vi "BuildCommand_InvokePPP.vi"(8 "error in (no error)":errorcluster, 11 "Cluster":T49 {"PersistentData"."RecircPumpFlow"."Recirc Pump Flow Set - R6" min=0.0 max=20.0; "PersistentData"."RecircPumpFlow"."Recirc Pump Flow Set - R5" min=0.0 max=20.0; "PersistentData"."RecircPumpFlow"."Recirc Pump Flow Set - R4" min=0.0 max=20.0; "PersistentData"."RecircPumpFlow"."Recirc Pump Flow Set - R3" min=0.0 max=20.0; "PersistentData"."RecircPumpFlow"."Recirc Pump Flow Set - R2" min=0.0 max=20.0; "PersistentData"."RecircPumpFlow"."Recirc Pump Flow Set - R1" min=0.0 max=20.0; "PersistentData"."MiniscusPressure"."Meniscus Pressure Set - R6" min=0.0 max=20.0; "PersistentData"."MiniscusPressure"."Meniscus Pressure Set - R5" min=0.0 max=20.0; "PersistentData"."MiniscusPressure"."Meniscus Pressure Set - R4" min=0.0 max=20.0; "PersistentData"."MiniscusPressure"."Meniscus Pressure Set - R3" min=0.0 max=20.0; "PersistentData"."MiniscusPressure"."Meniscus Pressure Set - R2" min=0.0 max=20.0; "PersistentData"."MiniscusPressure"."Meniscus Pressure Set - R1" min=0.0 max=20.0; "PersistentData"."Meniscus Vac Pump Speed" min=0.0 max=100.0}) -> (0 "error out":errorcluster, 2 "NextState":string, 3 "PPP Dithered Images":path[](array[path]))   [LabVIEW 2022 SP3, in "TopLevel.lvclass"]
uses:
  TopLevel.lvclass
  IO/IO.lvclass
  GIS Printer/GIS Printer.lvclass
  Motor Controller/Motor Controller.lvclass
  Typedefs/Digilens Config Cluster.ctl
  Typedefs/Motor Controller Config Data.ctl
  IO/Typedefs/IO Config Data.ctl
  IO/Typedefs/DCON_DeviceConfig--Cluster.ctl
  IO/Typedefs/Channel Data.ctl
  GIS Printer/Typedefs/PrinterConfiguration--Cluster.ctl
  DAQWFE/LV_Source/Subsystems/DAQ/DataTypes/TD DAQ Settings--cluster.ctl
  DAQWFE/LV_Source/Subsystems/DAQ/DataTypes/TD DI Instrument Settings--cluster.ctl
  DAQWFE/LV_Source/Subsystems/DAQ/DataTypes/TD AI Instrument Settings--cluster.ctl
  DAQWFE/LV_Source/Subsystems/DAQ/DataTypes/TD AI InstSettings--cluster.ctl
  DAQWFE/LV_Source/Subsystems/DAQ/Process/ProcessSupport/TD SimAI Ranges--cluster.ctl
  Common/Controls/DLPConfig_Initialization.ctl
  DLP2/DataTypes/DLP2_PrinterCompensationProperties.ctl
  DLP2/DataTypes/DLP2_PrinterHeadProperties.ctl
  Common/Controls/DLPConfig)Init_HeadPropertyAttr--Cluster.ctl
  DLP2/DataTypes/DLP2_PrinterMaterialProperties.ctl
  Typedefs/InkIdleNodeConfigXML--Cluster.ctl
  Typedefs/InkProcessNodeConfigXML--Cluster.ctl
  Motor Controller/Typedefs/Status.ctl
  Motor Controller/Typedefs/Stage Move Data.ctl
  Motor Controller/Typedefs/Batch Index Speed Data.ctl
  Motor Controller/Typedefs/Move Status.ctl
  IO/Typedefs/ICP1-D0 Channel Names.ctl
  IO/Typedefs/Pre Purge Parameters.ctl
  Typedefs/API Command Enum.ctl
  Database/Database.lvclass
  DLP2/DLP2.lvclass
  Common/Controls/TD MasterConfiguration DLPC2--cluster.ctl
  Common/Controls/DLPC2_Path--Cluster.ctl
  Common/Controls/TD HeadColorPaneMappingAll--cluster.ctl
  Common/Controls/TD HeadColorPaneMapping--cluster.ctl
  Typedefs/SpitVoltages--Cluster.ctl
  Typedefs/PrimingMode APIData.ctl
  Typedefs/PurgeMode--Enum.ctl
  Typedefs/PrinterHeads--Enum.ctl
  Common/Controls/RecipeInfo--Cluster.ctl
  DAQWFE/LV_Source/Subsystems/DAQ/DAQ.lvclass
  <vilib>/vision/Image Controls.llb/IMAQ Image.ctl
  Typedefs/TiffImageData--Cluster.ctl
  Common/Controls/Imageresolution--cluster.ctl
  GIS Printer/Typedefs/GIS Status--Cluster.ctl
  GIS Printer/Typedefs/HeadEnableStatus--cluster.ctl
  <vilib>/TELLC/Dynamic CVT API/TD Dynamic CVT DVR--ref.ctl
  DLP2/DataTypes/SeperateLayersPython--cluster.ctl
  Common/Controls/PythonVersion--Enum.ctl
  Common/Controls/PersistentData--Cluster.ctl
  Common/Controls/DLPConfig_RecipePrints.ctl
  Common/Controls/DLPConfig_CalibrationPrints.ctl
  Typedefs/LoginEventData--CLuster.ctl
  Typedefs/UserLevel--Enum.ctl
  Typedefs/printWeights--cluster.ctl
  DLP2/DataTypes/PPP_Python--cluster.ctl
  Common/Controls/DLP_MaterialToHeadMapping--Cluster.ctl
types:
  T1 = typedef "TopLevel.lvclass/Digilens Config Cluster.ctl" = cluster{"Motion Controller":T2, "IO Config":T3, "PrinterConfiguration":T6, "DAQ Settings":T7}
  T2 = typedef "Motor Controller.lvclass/Motor Controller Config Data.ctl" = cluster{"Motor IP Addresss":string, "Current Position":i32, "Pulse_Per_mm":i32, "PrePrint":dbl[], "Load Position_mm":i32, "Laminate Position_mm":i32}
  T3 = typedef "IO.lvclass/IO Config Data.ctl" = cluster{"DAQDevices":T4[], "DI Channels":T5[], "DO Channels":T5[], "Material Names":string[], "AI Channels":T5[], "AO Channels":T5[]}
  T4 = typedef "IO.lvclass/DCON_DeviceConfig--Cluster.ctl" = cluster{"COM":string, "DeviceName":string, "BaudRate":u32, "Number of Channels":i32, "DeviceAddress":i32, "Enable":bool}
  T5 = typedef "IO.lvclass/Channel Data.ctl" = cluster{"Channel Name":string, "Device Name":string, "Channel No":string}
  T6 = typedef "GIS Printer.lvclass/PrinterConfiguration--Cluster.ctl" = cluster{"IPAddress":string, "Move Stage on RTP Command?":bool, "Stage Move Position":string, "PH1-Prime Path":path, "PH2-Prime Path":path, "PH3-Prime Path":path, "PH4-Prime Path":path, "PH5-Prime Path":path, "PH6-Prime Path":path, "PrintScriptsFolder":path, "PurgeScriptsFolder":path, "StageScriptsFolder":path, "PH1-HeatOn Path":path, "PH2-HeatOn Path":path, "PH3-HeatOn Path":path, "PH4-HeatOn Path":path, "PH5-HeatOn Path":path, "PH6-HeatOn Path":path, "PH1-HeatOff Path":path, "PH2-HeatOff Path":path, "PH3-HeatOff Path":path, "PH4-HeatOff Path":path, "PH5-HeatOff Path":path, "PH6-HeatOff Path":path}
  T7 = typedef "DAQ.lvclass/TD DAQ Settings--cluster.ctl" = cluster{"Simulate DAQ":bool, "DI Settings":T8[], "AI Settings":T9[], "Relay IONames":string[], "AO IONames":string[], "AO NChan SingleTask":bool}
  T8 = typedef "DAQ.lvclass/TD DI Instrument Settings--cluster.ctl" = cluster{"Disable":bool, "DI TaskName":string, "DI RefreshIntv":i32}
  T9 = typedef "DAQ.lvclass/TD AI Instrument Settings--cluster.ctl" = cluster{"Disable":bool, "AI TaskName":string, "AI InstSettings":T10, "SimAI Ranges":T11}
  T10 = typedef "DAQ.lvclass/TD AI InstSettings--cluster.ctl" = cluster{"DaqRate":dbl, "NumSamples":i32}
  T11 = typedef "DAQ.lvclass/TD SimAI Ranges--cluster.ctl" = cluster{"lo":dbl, "hi":dbl}
  T12 = typedef "DLPConfig_Initialization.ctl" = cluster{"PrinterInitialization":cluster{"Printer":cluster{"#attributes":cluster{"Name":string}}, "VacPumpSet":cluster{"#attributes":cluster{"VacPumpEnable":bool, "VacPumpSpeed":dbl}}, "HIBEnable":cluster{"#attributes":cluster{"HIB1Enable":bool, "HIB2Enable":bool, "HIB3Enable":bool, "HIB4Enable":bool, "HIB5Enable":bool, "HIB6Enable":bool}}, "PrinterCompensation":T13}, "HeadSet":cluster{"HeadProperties":T14[]}, "InkSet":cluster{"Ink":T16[]}, "Troubleshooting":cluster{"PMBLogging":cluster{"#attributes":cluster{"PMBMonitorDuringPrint":bool, "PMBMonitorDuringIdle":bool, "LogSwatheInputData":bool, "LogSwatheOutputData":bool, "LogPrintheadColourPlanes":bool, "LogPMBCommunication":bool, "LogSimulatedOutput":bool, "LogAllPMBCommunicationData":bool, "LogPMBSpace":bool, "ExtendedPMBSpaceLogging":bool, "LogPMBWriteSpeed":bool, "LogUsbRetries":bool}}, "HIBLogging":cluster{"#attributes":cluster{"HIBMonitoringDuringPrint":bool, "HIBMonitoringLog":bool}}}}
  T13 = typedef "DLP2_PrinterCompensationProperties.ctl" = cluster{"#attributes":cluster{"AppName":string, "PrintWeightMultiplier":dbl, "Rotation":bool, "Driver":string, "Server":string, "Database":string, "User":string, "Password":string}}
  T14 = typedef "DLP2_PrinterHeadProperties.ctl" = cluster{"#attributes":T15}
  T15 = typedef "DLPConfig)Init_HeadPropertyAttr--Cluster.ctl" = cluster{"HeadNumber":u8, "Material":string, "HeadLocalX":dbl, "HeadLocalY":dbl, "HeadRotationAngle":dbl, "VH2L_Hi":dbl, "VH2R_Hi":dbl, "VH1LA_Hi":dbl, "VH1LB_Hi":dbl, "VH1RA_Hi":dbl, "VH1RB_Hi":dbl, "VH2L_Lo":dbl, "VH2R_Lo":dbl, "VH1LA_Lo":dbl, "VH1LB_Lo":dbl, "VH1RA_Lo":dbl, "VH1RB_Lo":dbl}
  T16 = typedef "DLP2_PrinterMaterialProperties.ctl" = cluster{"#attributes":cluster{"InkType":string, "PrePrintPurge":bool, "PurgeTime":dbl, "PurgeCount":i32, "Density":dbl, "NumberofDrops":i32, "PrintWeight":dbl, "PrintheadPrime":bool}, "Idle":T17, "Process":T18}
  T17 = typedef "InkIdleNodeConfigXML--Cluster.ctl" = cluster{"ShortIdle":cluster{"#attributes":cluster{"Heat":dbl, "Meniscus":dbl, "Recirculation":bool}}, "LongIdle":cluster{"#attributes":cluster{"Heat":dbl, "Meniscus":dbl, "Recirculation":bool}}}
  T18 = typedef "InkProcessNodeConfigXML--Cluster.ctl" = cluster{"C30_Process":cluster{"#attributes":cluster{"Heat":dbl, "Meniscus":dbl, "Recirculation":bool, "ColorPlane":string}}, "S30_Process":cluster{"#attributes":cluster{"Heat":dbl, "Meniscus":dbl, "Recirculation":bool, "ColorPlane":string}}}
  T19 = typedef "Motor Controller.lvclass/Status.ctl" = cluster{"Motor Controller Config Data":T2, "Motor Controller Data":cluster{"Enabled?":bool}, "Stage Move":T20, "Stage Busy?":bool}
  T20 = typedef "Motor Controller.lvclass/Stage Move Data.ctl" = cluster{"Current Step":string, "Move Data":T21[]}
  T21 = typedef "Motor Controller.lvclass/Batch Index Speed Data.ctl" = cluster{"Batch & Cycle":string, "Move":cluster{"Index_mm":i32, "Speed_mm_s":i32}, "Status":T22}
  T22 = typedef "Motor Controller.lvclass/Move Status.ctl" = enum16{"Pending", "In Progress", "Completed"}
  T23 = typedef "IO.lvclass/ICP1-D0 Channel Names.ctl" = enum16{"None", "Meniscus Pressure Reg PWR - R1", "Meniscus Pressure Reg PWR - R2", "Meniscus Pressure Reg PWR - R3", "Meniscus Pressure Reg PWR - R4", "Meniscus Pressure Reg PWR - R5", "Meniscus Pressure Reg PWR - R6", "Clear Stage Alarm", "Servo ON", "Purge Valve Open - R1", "Purge Valve Open - R2", "Purge Valve Open - R3", "Purge Valve Open - R4", "Purge Valve Open - R5", "Purge Valve Open - R6"}
  T24 = typedef "TopLevel.lvclass/Pre Purge Parameters.ctl" = cluster{"GIS File Path":path, "Duration (s)":dbl, "No. of Repeats":i32}
  T25 = typedef "TopLevel.lvclass/API Command Enum.ctl" = enum16{"Execute Printer Commands", "Pre Purge", "Enable Ink Ch-1", "Enable Ink Ch-2", "Enable Ink Ch-3", "Enable Ink Ch-4", "Enable Ink Ch-5", "Enable Ink Ch-6", "Disable Ink Ch-1", "Disable Ink Ch-2", "Disable Ink Ch-3", "Disable Ink Ch-4", "Disable Ink Ch-5", "Disable Ink Ch-6", "ExecuteIdlePrintCycle", "StopIdlePrintCycle", "Abort", "LoadDLP2GUIConfig", "SaveDLP2GUIConfig", "PrimingMode", "SetHeadTemperature", "EnableHead", "EnableHeadHeat", "SetSystemMode", "HeadPrint", "AbortAll", "Send Printer String", "WriteInitXML"}
  T26 = typedef "TD MasterConfiguration DLPC2--cluster.ctl" = cluster{"Paths":T27, "ColorPaneMapping":T28, "Materials":string[], "ColorPlanes":string[], "SpitVoltages_Half":T30, "SpitVoltages_Full":T30, "SystemMode":string[], "PrimeModeConfig":T31[], "Running Average Duration_s":dbl}
  T27 = typedef "DLPC2_Path--Cluster.ctl" = cluster{"DigiBit WG Design Folder":path, "Compensated GS Image Folder":path, "Nozzle GS Files Head 1":path, "Nozzle GS Files Head 2":path, "Nozzle GS Files Head 3":path, "Nozzle GS Files Head 4":path, "Nozzle GS Files Head 5":path, "Nozzle GS Files Head 6":path}
  T28 = typedef "TD HeadColorPaneMappingAll--cluster.ctl" = cluster{"Head 1":T29, "Head 2":T29, "Head 3":T29, "Head 4":T29, "Head 5":T29, "Head 6":T29}
  T29 = typedef "TD HeadColorPaneMapping--cluster.ctl" = cluster{"Material":string, "ColorPane":string}
  T30 = typedef "SpitVoltages--Cluster.ctl" = cluster{"1":dbl, "2":dbl, "3":dbl, "4":dbl, "5":dbl, "6":dbl}
  T31 = typedef "TopLevel.lvclass/PrimingMode APIData.ctl" = cluster{"Interval (s)":dbl, "PurgeDuration (s)":dbl, "Repeats":u8, "PrimingMode":T32, "Head":T33, "Frequency (Hz)":i32, "PrintWeight":dbl}
  T32 = typedef "PurgeMode--Enum.ctl" = enum16{"Pre-Purge", "Purge", "Spit", "Shake"}
  T33 = typedef "PrinterHeads--Enum.ctl" = enum16{"-1", "1", "2", "3", "4", "5", "6"}
  T34 = typedef "RecipeInfo--Cluster.ctl" = cluster{"Path":path, "Type":string, "Product":string}
  T35 = typedef "IMAQ Image.ctl" = refnum<image>
  T36 = typedef "TiffImageData--Cluster.ctl" = cluster{"ImageBufferMain":u8[][], "ChannelTargetMaterials":string[], "MaterialNames":string[]}
  T37 = typedef "Imageresolution--cluster.ctl" = cluster{"X Resolution":i32, "Y Resolution":i32}
  T38 = typedef "GIS Status--Cluster.ctl" = cluster{"HeadEnabled":bool, "SpitEnabled":bool, "HeaterEnabled":bool, "TargetTemperature":dbl, "CurrentTemperature":dbl}
  T39 = typedef "HeadEnableStatus--cluster.ctl" = cluster{"PH1_Enable":bool, "PH2_Enable":bool, "PH3_Enable":bool, "PH4_Enable":bool, "PH5_Enable":bool, "PH6_Enable":bool}
  T40 = typedef "TD Dynamic CVT DVR--ref.ctl" = refnum<data-value>
  T41 = typedef "SeperateLayersPython--cluster.ctl" = cluster{"Path_to_Tiff":path, "OutputFolder":path, "DPI_x":i32, "DPI_y":i32, "Python_Version":T42}
  T42 = typedef "PythonVersion--Enum.ctl" = enum16{"3.9 64", "3.9 32", "3.12 64", "3.12 32"}
  T43 = typedef "PersistentData--Cluster.ctl" = cluster{"ToolIdle":bool, "Meniscus Vac Pump Speed":dbl, "InkChEnable":cluster{"Enable Ink Ch-1":bool, "Enable Ink Ch-2":bool, "Enable Ink Ch-3":bool, "Enable Ink Ch-4":bool, "Enable Ink Ch-5":bool, "Enable Ink Ch-6":bool}, "HeatEnable":cluster{"Heater-1 Off":bool, "Heater-2 Off":bool, "Heater-3 Off":bool, "Heater-4 Off":bool, "Heater-5 Off":bool, "Heater-6 Off":bool}, "MiniscusPressure":cluster{"Meniscus Pressure Set - R1":dbl, "Meniscus Pressure Set - R2":dbl, "Meniscus Pressure Set - R3":dbl, "Meniscus Pressure Set - R4":dbl, "Meniscus Pressure Set - R5":dbl, "Meniscus Pressure Set - R6":dbl}, "RecircPumpFlow":cluster{"Recirc Pump Flow Set - R1":dbl, "Recirc Pump Flow Set - R2":dbl, "Recirc Pump Flow Set - R3":dbl, "Recirc Pump Flow Set - R4":dbl, "Recirc Pump Flow Set - R5":dbl, "Recirc Pump Flow Set - R6":dbl}}
  T44 = typedef "DLPConfig_RecipePrints.ctl" = cluster{"CellPrintRecipe":cluster{"#attributes":cluster{"Type":string, "RecipeName":string, "Product":string}, "CellPrint":cluster{"#attributes":cluster{"PrintImageFile":string, "PrintPass":i32, "PrintMode":string, "EncoderSource":string, "PrintGoSource":string, "DitheredSavePath":string, "GSSavePath":string}}[], "InkCompensationSet":cluster{"InkCompensation":cluster{"#attributes":cluster{"InkType":string, "Waveform":string, "ZoneCompensation":bool, "ZoneCompFile":string, "Overprint":dbl, "Bitmap":string, "SaveGSImg":bool, "GSSource":string, "GSValFile":string}}[]}}}
  T45 = typedef "DLPConfig_CalibrationPrints.ctl" = cluster{"CellPrintRecipe":cluster{"#attributes":cluster{"Type":string, "RecipeName":string, "Product":string}, "CellPrint":cluster{"#attributes":cluster{"PrintImageFile":string, "PrintPass":i32, "EncoderSource":string, "PrintGoSource":string, "Head":i32}}[], "InkCompensationSet":cluster{"InkCompensation":cluster{"#attributes":cluster{"InkType":string, "Waveform":string, "ZoneCompensation":bool}}[]}}}
  T46 = typedef "LoginEventData--CLuster.ctl" = cluster{"UserLevel":T47, "Login Time":timestamp}
  T47 = typedef "UserLevel--Enum.ctl" = enum16{"None", "Operator", "Engineer"}
  T48 = typedef "printWeights--cluster.ctl" = cluster{"Weights 1":dbl, "Weights 2":dbl, "Weights 3":dbl, "Weights 4":dbl, "Weights 5":dbl, "Weights 6":dbl}
  T49 = cluster{"Core":cluster{"Current VI Reference":refnum<vi>, "Close Panel on Exit?":bool}, "IO":refnum<class "IO.lvclass">, "GIS Printer":refnum<class "GIS Printer.lvclass">, "Motor Controller":refnum<class "Motor Controller.lvclass">, "Methods:Accessors:Digilens Config":T1, "Methods:Accessors:PrinterInitializationXML":T12, "Status":T19, "Exit Event":refnum<user-event>, "Purge\\PrePurge Channel Name":T23, "Pre Purge Parameters":T24, "API Command":T25, "TopLevel out":refnum<class "TopLevel.lvclass">, "Database":refnum<class "Database.lvclass">, "DLP2":refnum<class "DLP2.lvclass">, "DLP2Config":T26, "Materials":string[], "Color Panes":string[], "ConfigSaveRequired":bool, "DLP2ConfigLoaded":T26, "PrintDesign":T34, "DAQ":refnum<class "DAQ.lvclass">, "RGB Image":T35, "Planes Image":T35, "TIFFImageData":T36, "Image Resolution":T37, "Pre Purge API Data":T31, "Prime Names":cluster{"Prime 1":string, "Prime 2":string, "Prime 3":string, "Prime 4":string, "Prime 5":string, "Prime 6":string}, "Heater Enable":cluster{"HeaterEnblHead":T33, "Enable":bool}, "Head Temp ":cluster{"Head 1":cluster{"Actual":dbl, "Target":dbl}, "Head 2":cluster{"Actual":dbl, "Target":dbl}, "Head 3":cluster{"Actual":dbl, "Target":dbl}, "Head 4":cluster{"Actual":dbl, "Target":dbl}, "Head 5":cluster{"Actual":dbl, "Target":dbl}, "Head 6":cluster{"Actual":dbl, "Target":dbl}}, "GISHeadStatus":T38[], "SettingsUpdate":variant, "HeadStatus":T39, "Methods:Accessors:ConfigDict":T40, "Print":cluster{"RecipeXMLPath":path}, "SeparateLayers":T41, "PersistentData":T43, "HeadStatusPollData":T39, "CurrentDLPRecipe":T44, "CalibrationPrints":T45, "Login":T46, "PrintWeights":T48, "PrePrimeDone":bool, "PrePrimeTmrEnabled":bool, "PPP_Ditherered_Images":path[]}
  T50 = cluster{"AppName":string, "PrintWeightMultiplier":dbl, "Rotation":bool, "Driver":string, "Server":string, "Database":string, "User":string, "Password":string}
  T51 = cluster{"#attributes":cluster{"PrintImageFile":string, "PrintPass":i32, "PrintMode":string, "EncoderSource":string, "PrintGoSource":string, "DitheredSavePath":string, "GSSavePath":string}}[]
  T52 = cluster{"#attributes":cluster{"InkType":string, "Waveform":string, "ZoneCompensation":bool, "ZoneCompFile":string, "Overprint":dbl, "Bitmap":string, "SaveGSImg":bool, "GSSource":string, "GSValFile":string}}[]
  T53 = cluster{"#attributes":cluster{"PrintImageFile":string, "PrintPass":i32, "PrintMode":string, "EncoderSource":string, "PrintGoSource":string, "DitheredSavePath":string, "GSSavePath":string}}
  T54 = typedef "PPP_Python--cluster.ctl" = cluster{"product":string, "printer":string, "printhead":T33, "material":string, "weight":dbl, "density":dbl, "overprint":dbl, "print_wt_multiplier":dbl, "num_of_drops":i32, "gs_source":string, "gs_val_file":path, "zone_compensation":bool, "zone_comp_file":path, "bitmap":path, "save_gs_img":bool, "dithered_save_path":path, "gs_save_path":path, "rotation":bool, "driver":string, "server":string, "database":string, "user":string, "password":string}
  T55 = typedef "DLP_MaterialToHeadMapping--Cluster.ctl" = cluster{"Head":u8, "Ink":T16}
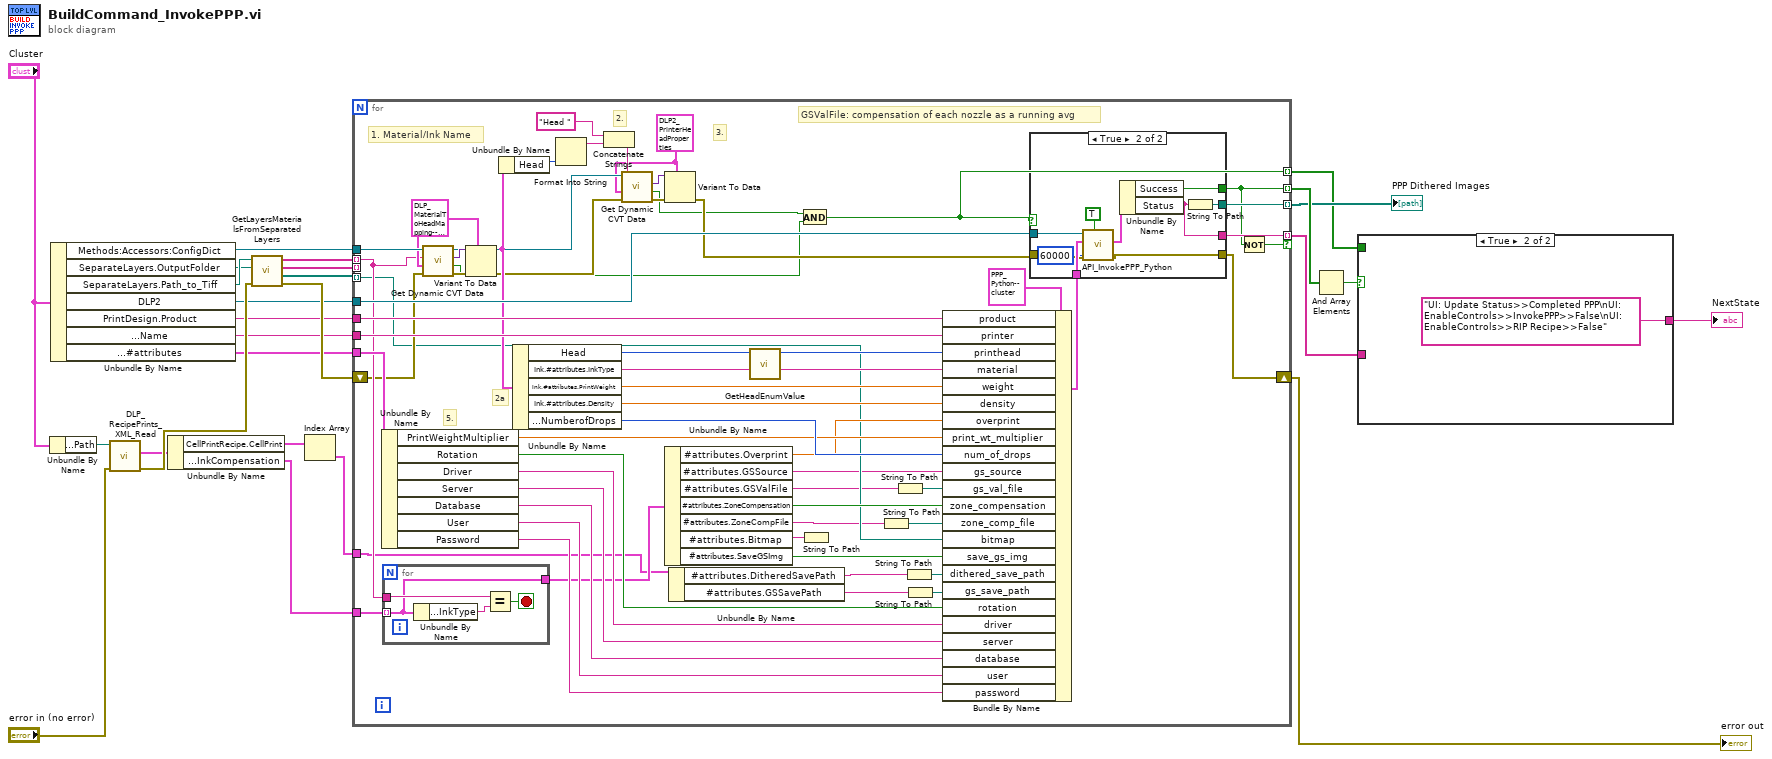
[diagram p0: block diagram]
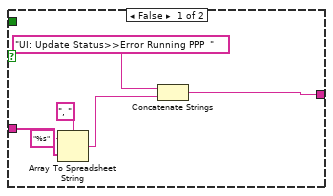
[diagram p2: hidden frame]
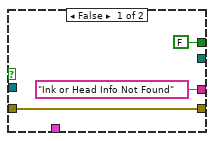
[diagram p3: hidden frame]
diagram:
  n1 = Unbundle By Name("Cluster") -> ("PrintDesign.Path"=w10:path)
  n2 = Unbundle By Name("Cluster") -> ("Methods:Accessors:ConfigDict"=w7:T40, "SeparateLayers.OutputFolder"=w4:path, "SeparateLayers.Path_to_Tiff"=w5:path, "DLP2"=w2:refnum<class "DLP2.lvclass">, "PrintDesign.Product"=w3:string, "Methods:Accessors:PrinterInitializationXML.PrinterInitialization.Printer.#attributes.Name"=w1:string, "Methods:Accessors:PrinterInitializationXML.PrinterInitialization.PrinterCompensation.#attributes"=w9:T50)
  n3 = call "DLP_RecipePrints_XML_Read.vi"("error in (no error)"="error in (no error)", "Recipe XML File Path"=w10) -> ("error out"=w25:errorcluster, "DLPRecipe"=w12:T44)  [unwired: 8 in]
  n4 = Unbundle By Name(w12) -> ("CellPrintRecipe.CellPrint"=w17:T51, "CellPrintRecipe.InkCompensationSet.InkCompensation"=w13:T52)
  n5 = call "GetLayersMaterialsFromSeparatedLayers.vi"("error in (no error)"=w25, "OutputFolder"=w4, "Path_to_Tiff"=w5) -> ("error out"=w15:errorcluster, "LayerNo"=w8:string[], "Materials"=w6:string[], "Separated Layer bmp []"=w16:path[])  [unwired: 4 in, 1 out]
  n6 = Index Array(array=w17) -> (element=w18:T53)  [unwired: 1 in]
  n7 = for {
    tunnel: w1 -> [w85]
    tunnel: w2 -> [w83]
    tunnel: w3 -> [w82]
    tunnel: w6 -> [w65] mode=indexing
    tunnel: w7 -> [w81]
    tunnel: w8 -> [_] mode=indexing
    tunnel: w9 -> [w74]
    tunnel: w13 -> [w66]
    shift-right: [w45] -> w26
    shift-left: w15 -> [w47]
    tunnel: [w39] -> w19 mode=indexing
    tunnel: w16 -> [w37] mode=indexing
    tunnel: w18 -> [w36]
    tunnel: [w30] -> w21 mode=indexing
    tunnel: [w28] -> w22 mode=indexing
    tunnel: [w29] -> w24 mode=indexing if=w27
    w42 = T14 {"#attributes"={"HeadNumber"=0, "Material"="", "HeadLocalX"=0.0, "HeadLocalY"=0.0, "HeadRotationAngle"=0.0, "VH2L_Hi"=0.0, "VH2R_Hi"=0.0, "VH1LA_Hi"=0.0, "VH1LB_Hi"=0.0, "VH1RA_Hi"=0.0, "VH1RB_Hi"=0.0, "VH2L_Lo"=0.0, "VH2R_Lo"=0.0, "VH1LA_Lo"=0.0, "VH1LB_Lo"=0.0, "VH1RA_Lo"=0.0, "VH1RB_Lo"=0.0}}
    w77 = T55 {"Head"=0, "Ink"={"#attributes"={"InkType"="", "PrePrintPurge"=FALSE, "PurgeTime"=0.0, "PurgeCount"=0, "Density"=0.0, "NumberofDrops"=0, "PrintWeight"=0.0, "PrintheadPrime"=FALSE}, "Idle"={"ShortIdle"={"#attributes"={"Heat"=0.0, "Meniscus"=0.0, "Recirculation"=FALSE}}, "LongIdle"={"#attributes"={"Heat"=0.0, "Meniscus"=0.0, "Recirculation"=FALSE}}}, "Process"={"C30_Process"={"#attributes"={"Heat"=0.0, "Meniscus"=0.0, "Recirculation"=FALSE, "ColorPlane"=""}}, "S30_Process"={"#attributes"={"Heat"=0.0, "Meniscus"=0.0, "Recirculation"=FALSE, "ColorPlane"=""}}}}}
    # "GSValFile: compensation of each nozzle as a running avg"
    # "5."
    # "4."
    # "3."
    # "2a"
    # "2."
    # "1. Material/Ink Name"
    n8 = Unbundle By Name(w74) -> ("PrintWeightMultiplier"=w73:dbl, "Rotation"=w72:bool, "Driver"=w71:string, "Server"=w70:string, "Database"=w69:string, "User"=w68:string, "Password"=w67:string)
    n9 = for {
      tunnel: w66 -> [w101] mode=indexing
      tunnel: w65 -> [w103]
      tunnel: [w101] -> w64
      stop <- w102 stop-if-true
      n10 = Unbundle By Name(w101) -> ("#attributes.InkType"=w104:string)
      n11 = Equal?(x=w103, y=w104) -> (x = y?=w102:bool)
    }
    n12 = call <vilib>:"Get Dynamic CVT Data.vi"("error in (no error)"=w47, "default value (empty variant)"=w77, "DataName"=w65, "dCVT DVR"=w81) -> ("error out"=w80:errorcluster, "found"=w40:bool, "value"=w79:variant, "dCVT DVR out"=w51:T40)  [unwired: 4 in]
    n13 = Variant To Data(error in=w80, type=w77, Variant=w79) -> (data=w50:T55, error out=w48:errorcluster)
    n14 = Unbundle By Name(w50) -> ("Head"=w49:u8)
    n15 = Unbundle By Name(w50) -> ("Head"=w44:u8, "Ink.#attributes.InkType"=w84:string, "Ink.#attributes.PrintWeight"=w78:dbl, "Ink.#attributes.Density"=w76:dbl, "Ink.#attributes.NumberofDrops"=w75:i32)
    n16 = Format Into String(w49) -> (resulting string=w55:string)  [unwired: 3 in, 1 out]
    n17 = Concatenate Strings("Head " ("string"), w55) -> (w52:string)
    n18 = call <vilib>:"Get Dynamic CVT Data.vi"("error in (no error)"=w48, "default value (empty variant)"=w42, "DataName"=w52, "dCVT DVR"=w51) -> ("error out"=w53:errorcluster, "found"=w41:bool, "value"=w54:variant)  [unwired: 4 in, 1 out]
    n19 = Variant To Data(error in=w53, type=w42, Variant=w54) -> (error out=w46:errorcluster)  [unwired: 1 out]
    n20 = Unbundle By Name(w64) -> ("#attributes.Overprint"=w57:dbl, "#attributes.GSSource"=w31:string, "#attributes.GSValFile"=w32:string, "#attributes.ZoneCompensation"=w61:bool, "#attributes.ZoneCompFile"=w33:string, "#attributes.Bitmap"=w38:string, "#attributes.SaveGSImg"=w60:bool)
    n21 = Unbundle By Name(w36) -> ("#attributes.DitheredSavePath"=w35:string, "#attributes.GSSavePath"=w34:string)
    n22 = call "GetHeadEnumValue.vi"("Head"=w44) -> ("Head"=w43:T33)  [unwired: 9 in, 1 out]
    n23 = And(x=w41, y=w40) -> (x .and. y?=w39:bool)
    n24 = String To Path(string=w38) -> ()  [unwired: 1 out]
    n25 = String To Path(string=w33) -> (path=w62:path)
    n26 = String To Path(string=w32) -> (path=w63:path)
    n27 = String To Path(string=w35) -> (path=w59:path)
    n28 = String To Path(string=w34) -> (path=w58:path)
    n29 = Bundle By Name(cluster=T54 {"product"="", "printer"="", "printhead"=enum."1", "material"="", "weight"=0.0, "density"=0.0, "overprint"=0.0, "print_wt_multiplier"=0.0, "num_of_drops"=0, "gs_source"="", "gs_val_file"=path "", "zone_compensation"=FALSE, "zone_comp_file"=path "", "bitmap"=path "", "save_gs_img"=FALSE, "dithered_save_path"=path "", "gs_save_path"=path "", "rotation"=FALSE, "driver"="", "server"="", "database"="", "user"="", "password"=""} ("PPP_parameters"), "product"=w82, "printer"=w85, "printhead"=w43, "material"=w84, "weight"=w78, "density"=w76, "overprint"=w57, "print_wt_multiplier"=w73, "num_of_drops"=w75, "gs_source"=w31, "gs_val_file"=w63, "zone_compensation"=w61, "zone_comp_file"=w62, "bitmap"=w37, "save_gs_img"=w60, "dithered_save_path"=w59, "gs_save_path"=w58, "rotation"=w72, "driver"=w71, "server"=w70, "database"=w69, "user"=w68, "password"=w67) -> (w86:T54)
    n30 = case shown="True" w39 {
      tunnel: w86 -> [_ w100]
      tunnel: w83 -> [_ w99]
      tunnel: w46 -> [w90 w98]
      tunnel: [w90 w97] -> w45
      tunnel: [_ w93] -> w30
      tunnel: [FALSE ("Success") w92] -> w28
      tunnel: ["Ink or Head Info Not Found" ("Status") w91] -> w29
      frame False {
      }
      frame True {
        n31 = call "API_InvokePPP_Python.vi"("Timeout (ms)"=u32 60000, "Wait (F)"=TRUE, "error in (no error)"=w98, "PPP_parameters"=w100, "DLP2 in"=w99) -> ("error out"=w97:errorcluster, "Cluster"=w94:cluster{"Success":bool, "Status":string})  [unwired: 4 in, 1 out]
        n32 = Unbundle By Name(w94) -> ("Success"=w92:bool, "Status"=w91:string)
        n33 = String To Path(string=w91) -> (path=w93:path)
      }
    }
    n34 = Not(x=w28) -> (.not. x?=w27:bool)
  }
  "error out" <- w26
  "PPP Dithered Images" <- w21
  n35 = And Array Elements(Boolean array=w22) -> (logical AND=w23:bool)
  n36 = case shown="True" w23 {
    tunnel: [w107 "UI: Update Status>>Completed PPP\nUI: EnableControls>>InvokePPP>>False\nUI: EnableControls>>RIP Recipe>>False" ("DictName")] -> w20
    tunnel: w19 -> [_ _]
    tunnel: w24 -> [w109 _]
    frame False {
      n37 = Array To Spreadsheet String(delimiter (Tab)=", ", array=w109, 3:"%s" ("format string")) -> (spreadsheet string=w106:string)
      n38 = Concatenate Strings("UI: Update Status>>Error Running PPP  " ("DictName"), w106) -> (w107:string)
    }
    frame True {
    }
  }
  "NextState" <- w20
